vi "merlinGetFrequency.vi"(8 "error in":errorcluster, 11 "Port":refnum<visa-resource-name>) -> (0 "error out":errorcluster, 2 "Freq":string, 3 "Port out":refnum<visa-resource-name>)   [LabVIEW 2018]
panel:
  in  "Freq":u32
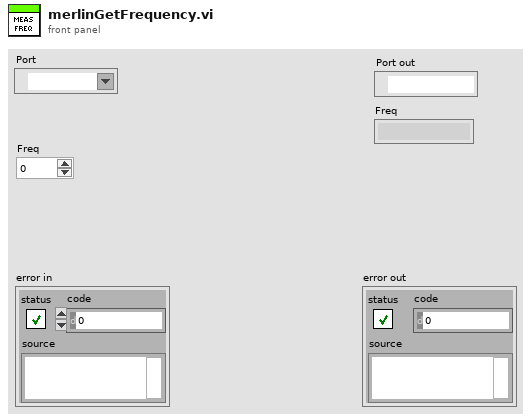
[diagram p1: front panel]
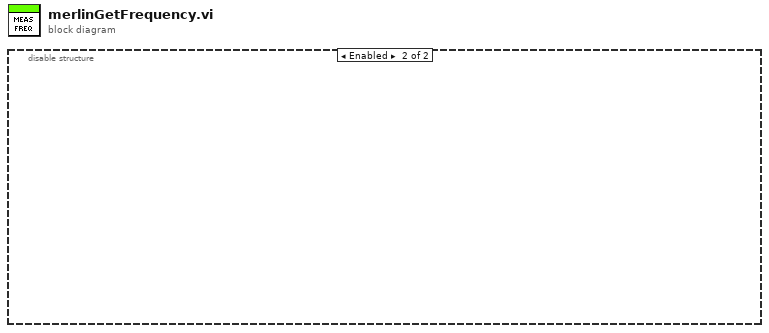
[diagram p0: block diagram]
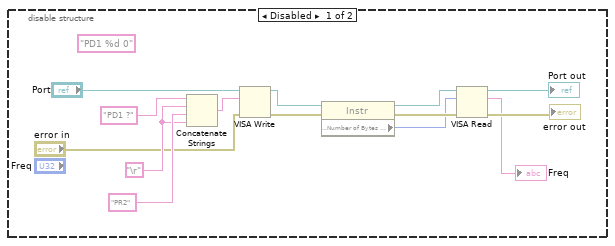
[diagram p2: hidden frame]
diagram:
  n1 = disable-structure shown="Enabled" {
    frame Disabled {
      w11 = "\r"
      (unwired) "PD1 %d 0" ("concatenated string")
      n2 = Concatenate Strings("PD1 ?" ("concatenated string"), w11, "PR2" ("concatenated string"), w11) -> (w13:string)
      n3 = VISA Write(VISA resource name="Port", write buffer=w13, error in (no error)="error in") -> (VISA resource name out=w8:refnum<visa-resource-name>, error out=w7:errorcluster)  [unwired: 1 out]
      n4 = property class="Instr"(reference=w8, error in=w7) -> (reference out=w5:refnum<visa-resource-name>, error out=w6:errorcluster, "Serial Settings:Number of Bytes at Serial Port"=w4:u32)
      n5 = VISA Read(VISA resource name=w5, byte count=w4, error in (no error)=w6) -> (VISA resource name out=→"Port out":refnum<visa-resource-name>, read buffer=→"Freq":string, error out=→"error out":errorcluster)  [unwired: 1 out]
    }
    frame Enabled {
    }
  }
